vi "getWFMQueueStatus.vi"(8 "error in (no error)":errorcluster, 10 "instance":string, 11 "DAQmx in":refnum<class "DAQmx.lvclass">) -> (0 "error out":errorcluster, 1 "Min AO Queue Filled":bool, 2 "AO queue #":i32, 3 "DAQmx out":refnum<class "DAQmx.lvclass">)   [LabVIEW 2019, in "DAQmx.lvclass"]
uses:
  DAQmx.lvclass
  DAQmx.lvclass/DAQmx.ctl
panel:
  out "Queue Chart":T1(graph)
  out "REF Y queue #":i32
  out "REF X queue #":i32
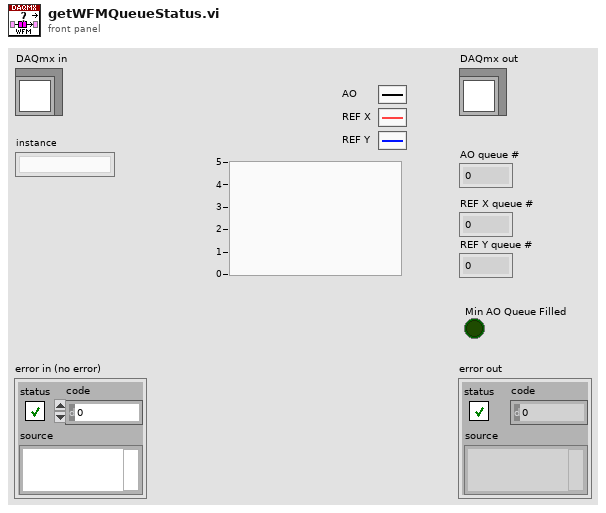
[diagram p1: front panel]
types:
  T1 = cluster{"# elements in queue":i32, "# elements in queue":i32, "# elements in queue":i32}
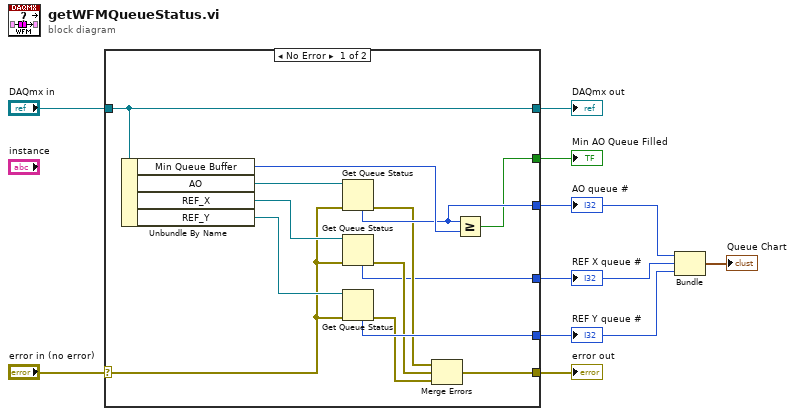
[diagram p0: block diagram]
diagram:
  n1 = case shown="No Error" "error in (no error)" {
    selector: "error in (no error)" -> [w15 w25]
    tunnel: [w19 w25] -> w8
    tunnel: [w23 w24] -> w6
    tunnel: "DAQmx in" -> [w23 w24]
    tunnel: [w16 _] -> w1
    tunnel: [w10 _] -> w5
    tunnel: [w11 _] -> w4
    tunnel: [w18 _] -> w3
    frame No Error {
      n2 = Unbundle By Name(w23) -> ("Min Queue Buffer"=w17:i32, "AO"=w22:refnum<queue>, "REF_X"=w21:refnum<queue>, "REF_Y"=w20:refnum<queue>)
      n3 = Get Queue Status(queue=w22, error in (no error)=w15) -> (error out=w13:errorcluster, # elements in queue=w16:i32)  [unwired: 1 in, 6 out]
      n4 = Get Queue Status(queue=w21, error in (no error)=w15) -> (error out=w14:errorcluster, # elements in queue=w11:i32)  [unwired: 1 in, 6 out]
      n5 = Get Queue Status(queue=w20, error in (no error)=w15) -> (error out=w12:errorcluster, # elements in queue=w18:i32)  [unwired: 1 in, 6 out]
      n6 = Merge Errors(w13, w14, w12) -> (w19:errorcluster)
      n7 = Greater Or Equal?(x=w16, y=w17) -> (x >= y?=w10:bool)
    }
    frame Error {
    }
  }
  "error out" <- w8
  "DAQmx out" <- w6
  "AO queue #" <- w1
  "Min AO Queue Filled" <- w5
  "REF X queue #" <- w4
  "REF Y queue #" <- w3
  n8 = Bundle("# elements in queue"=w1, "# elements in queue"=w4, "# elements in queue"=w3) -> (→"Queue Chart":T1)  [unwired: 1 in]
